vi "Graphics-Delete Plot.vi"(0 "XYGraph in":refnum<vi>, 9 "index":i32, 11 "error in (no error)":errorcluster) -> (4 "XYGraph out":refnum<vi>, 15 "error out":errorcluster)   [LabVIEW 2020]
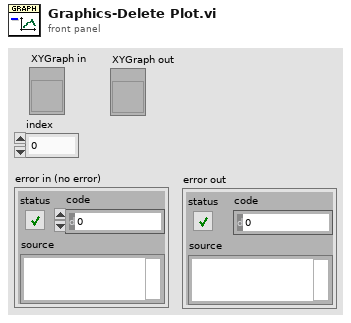
[diagram p1: front panel]
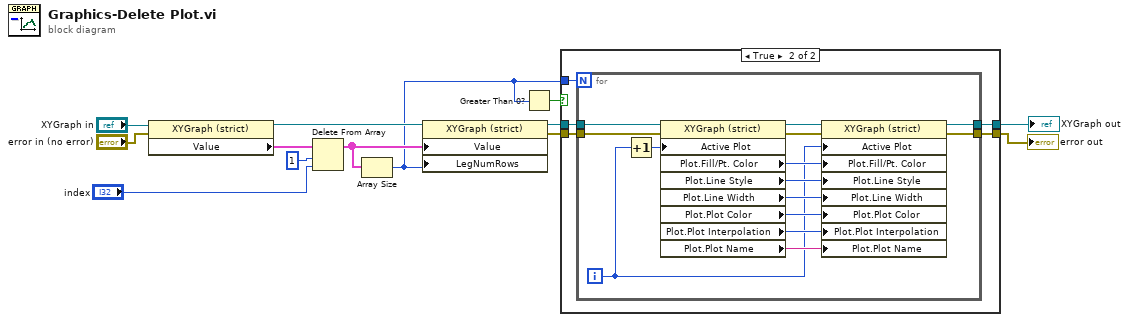
[diagram p0: block diagram]
diagram:
  n1 = property class="XYGraph (strict)"(reference="XYGraph in", error in="error in (no error)") -> (reference out=w13:refnum<vi>, "Value"=w6:cluster{"Frequency":dbl[], "Frequency":dbl[]}[])  [unwired: 1 out]
  n2 = Delete From Array(array=w6, length=1, index="index") -> (array with subset deleted=w3:cluster{"Frequency":dbl[], "Frequency":dbl[]}[])  [unwired: 1 out]
  n3 = Array Size(array=w3) -> (size(s)=w2:i32)
  n4 = property class="XYGraph (strict)"(reference=w13, "Value"=w3, "LegNumRows"=w2) -> (reference out=w10:refnum<vi>, error out=w9:errorcluster)  [unwired: 1 in]
  n5 = Greater Than 0?(x=w2) -> (x > 0?=w1:bool)
  n6 = case shown="True" w1 {
    tunnel: w10 -> [w15 w20]
    tunnel: w9 -> [w14 w19]
    tunnel: [w15 w18] -> w8
    tunnel: [w14 w17] -> w7
    tunnel: w2 -> [_ w16]
    frame False {
    }
    frame True {
      n7 = for {
        N: w16 -> [_]
        tunnel: w20 -> [w23]
        tunnel: w19 -> [w34]
        tunnel: [w25] -> w18
        tunnel: [w24] -> w17
        i -> [w21]
        n8 = Increment(x=w21) -> (x+1=w22:i32)
        n9 = property class="XYGraph (strict)"(reference=w23, error in=w34, "Active Plot"=w22) -> (reference out=w33:refnum<vi>, error out=w32:errorcluster, "Plot.Fill/Pt. Color"=w31:u32, "Plot.Line Style"=w30:u8, "Plot.Line Width"=w29:u8, "Plot.Plot Color"=w28:u32, "Plot.Plot Interpolation"=w27:u8, "Plot.Plot Name"=w26:string)
        n10 = property class="XYGraph (strict)"(reference=w33, error in=w32, "Active Plot"=w21, "Plot.Fill/Pt. Color"=w31, "Plot.Line Style"=w30, "Plot.Line Width"=w29, "Plot.Plot Color"=w28, "Plot.Plot Interpolation"=w27, "Plot.Plot Name"=w26) -> (reference out=w25:refnum<vi>, error out=w24:errorcluster)
      }
    }
  }
  "error out" <- w7
  "XYGraph out" <- w8
